vi "PA Init.vi"(5 "FilterLevel":i32, 6 "UseZeroSet":u8, 7 "AutoZeroSet":u8, 9 "SamplingRate":i32, 10 "Channel":i32, 11 "DevHandle":i32) -> (3 "function return":i32)   [LabVIEW 2010, in "power_analyzer.lvlib"]
doc: "int WINAPI PA_Init(int DevHandle,int Channel,int SamplingRate,unsigned char AutoZeroSet,unsigned char UseZeroSet,int FilterLevel);"
uses:
  power_analyzer.lvlib
  USB2XXX/trunk/USB2XXX/USB2XXX/vs2010/Release/USB2XXX.dll
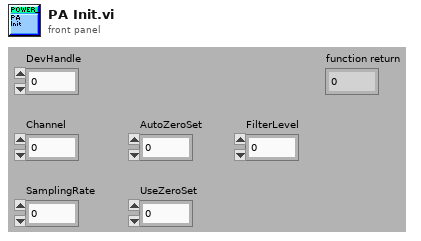
[diagram p1: front panel]
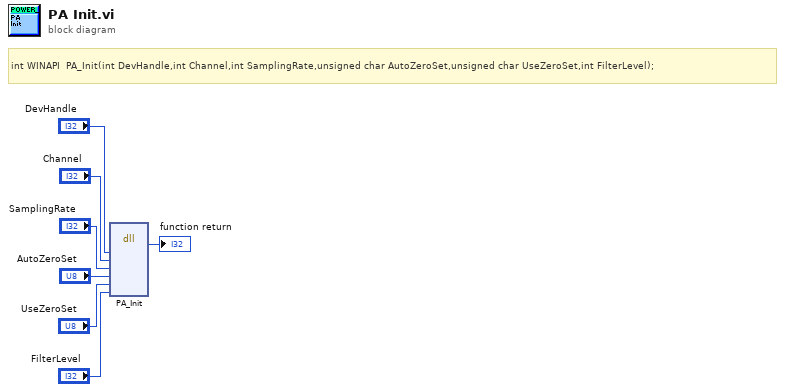
[diagram p0: block diagram]
diagram:
  # "int WINAPI  PA_Init(int DevHandle,int Channel,int SamplingRate,unsigned char AutoZeroSet,unsigned char UseZeroSet,int FilterLevel);"
  n1 = dll-call lib="E:/Projects/USB2XXX/trunk/USB2XXX/USB2XXX/vs2010/Release/USB2XXX.*" fn="PA_Init"("DevHandle"="DevHandle", "Channel"="Channel", "SamplingRate"="SamplingRate", "AutoZeroSet"="AutoZeroSet", "UseZeroSet"="UseZeroSet", "FilterLevel"="FilterLevel") -> (→"function return":i32)  [unwired: 9 in, 2 out]
